vi "Send Immediate Stop Msg.vi"(8 "error in (no error)":errorcluster, 11 "Message Enqueuer":refnum<class "Message Enqueuer.lvclass">) -> (0 "error out":errorcluster)   [LabVIEW 2017, in "PriorityStopMessage.lvclass"]
doc: "<License>\nCopyright © 2017 Composed Systems, LLC | All rights reserved\nwww.composed.io\n\nAuthor: Ethan Stern <ethan.stern@composed.io>\n\nThis software is provided \"AS IS\" WITHOUT WARRANTIES, either express or implied, AND IS FOR EDUCATIONAL PURPOSES ONLY.\n</License>"
uses:
  <vilib>/gpm_packages/@cs/actor-framework-messages/Source/PriorityStopMessage/PriorityStopMessage.lvclass
  <vilib>/ActorFramework/Message Enqueuer/Message Enqueuer.lvclass
  <vilib>/ActorFramework/Stop Msg/Stop Msg.lvclass
  C:/Program Files/National Instruments/LabVIEW 2017/vi.lib/ActorFramework/Message/Message.lvclass
  <vilib>/ActorFramework/Message Enqueuer/Message Priority.ctl
  <vilib>/ActorFramework/Message Enqueuer/Message Enqueuer.lvclass/Message Enqueuer.ctl
  <vilib>/ActorFramework/Message Priority Queue/Priority Enqueue.vi
panel:
  # "This method was not properly tested before pre-release!\nThe technique used here does not actually work and\nthere's no way around it with the current scoping of\nAF messaging resources. Your next best option is to use\nSend Priority Stop Msg with 'High' Priority."
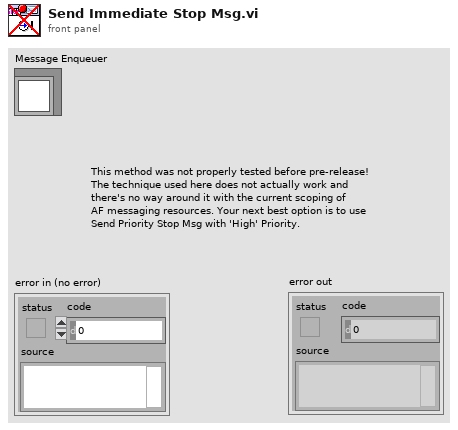
[diagram p1: front panel]
types:
  T1 = typedef "Actor Framework.lvlib/Message Enqueuer.lvclass/Message Priority.ctl" = enum16{"Low", "Normal", "High"}
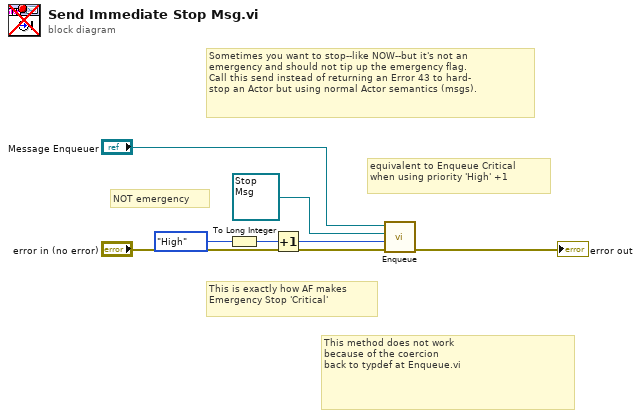
[diagram p0: block diagram]
diagram:
  # "This method does not work\nbecause of the coercion\nback to typdef at Enqueue.vi"
  # "equivalent to Enqueue Critical\nwhen using priority 'High' +1"
  # "This is exactly how AF makes\nEmergency Stop 'Critical'"
  # "NOT emergency"
  # "Sometimes you want to stop--like NOW--but it's not an\nemergency and should not tip up the emergency flag.\nCall this send instead of returning an Error 43 to hard-\nstop an Actor but using normal Actor semantics (msgs)."
  n1 = To Long Integer(number=Message_Priority."High" ("Message Priority (Normal)")) -> (32bit integer=w1:i32)
  n2 = Increment(x=w1) -> (x+1=w2:i32)
  n3 = call <vilib>:"Enqueue.vi"("error in (no error)"="error in (no error)", "Message Priority (Normal)"=w2, "Message"=refnum<class "Stop Msg.lvclass"> refnum ("Actor Framework:Stop Msg"), "Message Enqueuer in"="Message Enqueuer") -> ("error out"=→"error out":errorcluster)  [unwired: 6 in, 1 out]
